vi "Set Port.vi"(8 "error in (no error)":errorcluster, 10 "Port":u16, 11 "URI in":refnum<class "URI.lvclass">) -> (0 "error out":errorcluster, 3 "URI out":refnum<class "URI.lvclass">)   [LabVIEW 2020, in "Stream.lvlib" / "URI.lvclass"]
uses:
  URI.lvclass
  URI.lvclass/URI.ctl
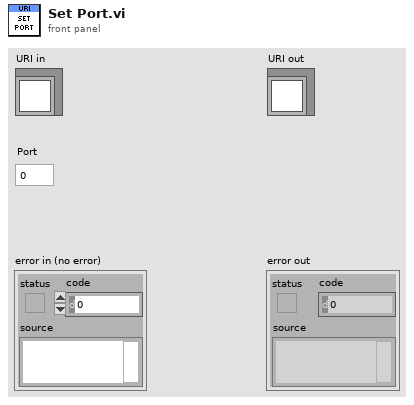
[diagram p1: front panel]
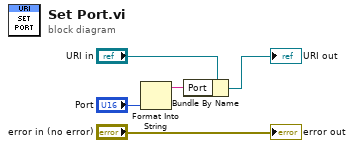
[diagram p0: block diagram]
diagram:
  n1 = Format Into String("Port") -> (resulting string=w1:string)  [unwired: 3 in, 1 out]
  n2 = Bundle By Name(cluster="URI in", "Port"=w1) -> (→"URI out":refnum<class "URI.lvclass">)
  "error out" <- "error in (no error)"
